vi "mca3test.vi"(0 "MCD #":i32) -> (1 "MCA-3 Data":u32[](graph), 2 "Spectrum Length":i32)   [LabVIEW 2013]
panel:
  out "MCA-3 Status":T1 {"Deadtime" format="%.2f"; "Livetime(Sweeps)" format="%.2f"; "NetSum" format="%.2f"; "TotalRate" format="%.2f"; "RoiSum" format="%.2f"; "TotalSum" format="%.2f"; "Realtime" format="%.2f"}
  out "MCA-3 Settings":T2 {"Dwellunit" format="%.0x"; "Prena" format="%.0x"; "Diguse" format="%.0x"; "LTimePreset" format="%.2f"; "SyncOut" format="%.0x"; "MCS Mode" format="%.0x"; "SweepPreset" format="%.2f"; "SaveData" format="%.0x"; "RTimepreset" format="%.2f"; "Roipreset" format="%.2f"}
  out "MCA3Dat Error":i32
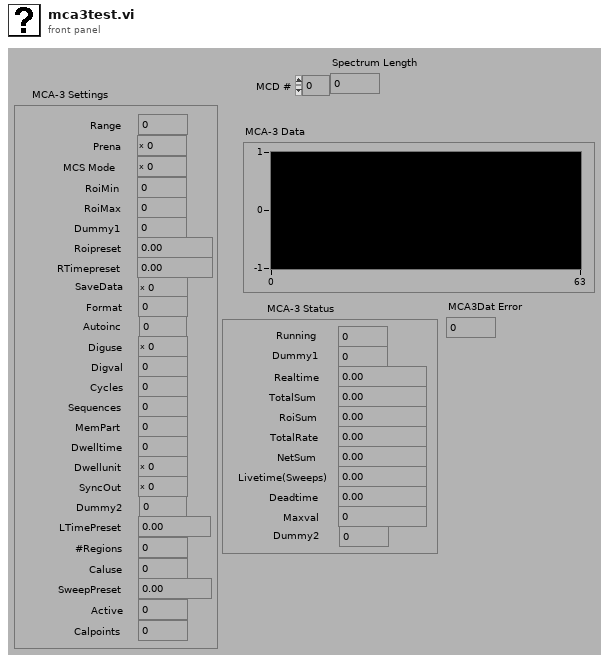
[diagram p1: front panel]
types:
  T1 = cluster{"Running":i32, "Dummy1":i32, "Realtime":dbl, "TotalSum":dbl, "RoiSum":dbl, "TotalRate":dbl, "NetSum":dbl, "Livetime(Sweeps)":dbl, "Deadtime":dbl, "Maxval":u32, "Dummy2":i32}
  T2 = cluster{"Range":i32, "Prena":u32, "MCS Mode":u32, "RoiMin":u32, "RoiMax":u32, "Dummy1":u32, "Roipreset":dbl, "RTimepreset":dbl, "SaveData":u32, "Format":i32, "Autoinc":i32, "Diguse":u32, "Digval":u32, "Cycles":u32, "Sequences":u32, "MemPart":u32, "Dwelltime":u32, "Dwellunit":u32, "SyncOut":u32, "Dummy2":u32, "LTimePreset":dbl, "#Regions":u32, "Caluse":u32, "SweepPreset":dbl, "Active":u32, "Calpoints":u32}
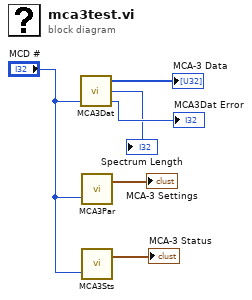
[diagram p0: block diagram]
diagram:
  n1 = call <userlib>:"MCA3Dat.vi"("MCD #"="MCD #") -> ("MCA3Dat Error"=→"MCA3Dat Error":i32, "Spectrum Length"=→"Spectrum Length":i32, "Data"=→"MCA-3 Data":u32[])  [unwired: 2 in]
  n2 = call <userlib>:"MCA3Par.vi"("MCD #"="MCD #") -> ("MCA-3 Settings"=→"MCA-3 Settings":T2)  [unwired: 1 in, 1 out]
  n3 = call <userlib>:"MCA3Sts.vi"("MCD #"="MCD #") -> ("MCA-3 Status"=→"MCA-3 Status":T1)  [unwired: 1 in, 1 out]
